vi "data collection.vi"(0 "Refnum in":T1, 1 "To Date":timestamp, 2 "Form Date":timestamp, 3 "Report filter":string, 5 "Shift":string, 7 "Select Line":string, 9 "Select Year":string, 11 "error in (no error)":errorcluster, 12 "columns":string[](array[string]), 13 "Select Month":string, 14 "table":string) -> (4 "Refnum out":T1, 6 "Table":string[][](array[string]), 8 "disabled index (col)":i32, 15 "error out":errorcluster)   [LabVIEW 2017]
uses:
  <vilib>/addons/database/Connection.llb/Conn ObjectReference.ctl
  <vilib>/addons/database/NI_Database_API.lvlib
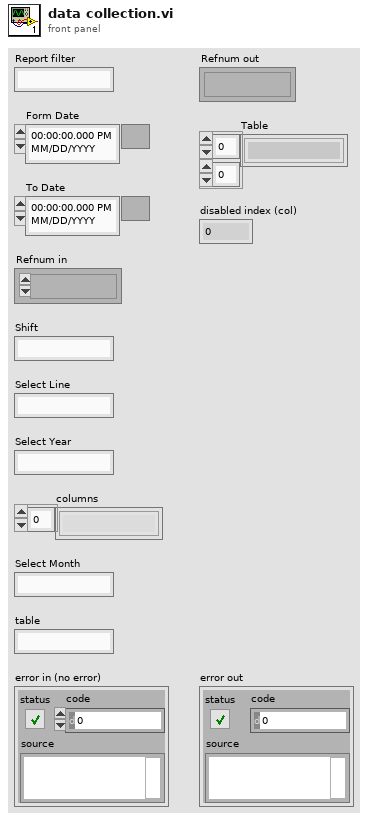
[diagram p1: front panel]
types:
  T1 = typedef "NI_Database_API.lvlib/Conn ObjectReference.ctl" = refnum<k1>
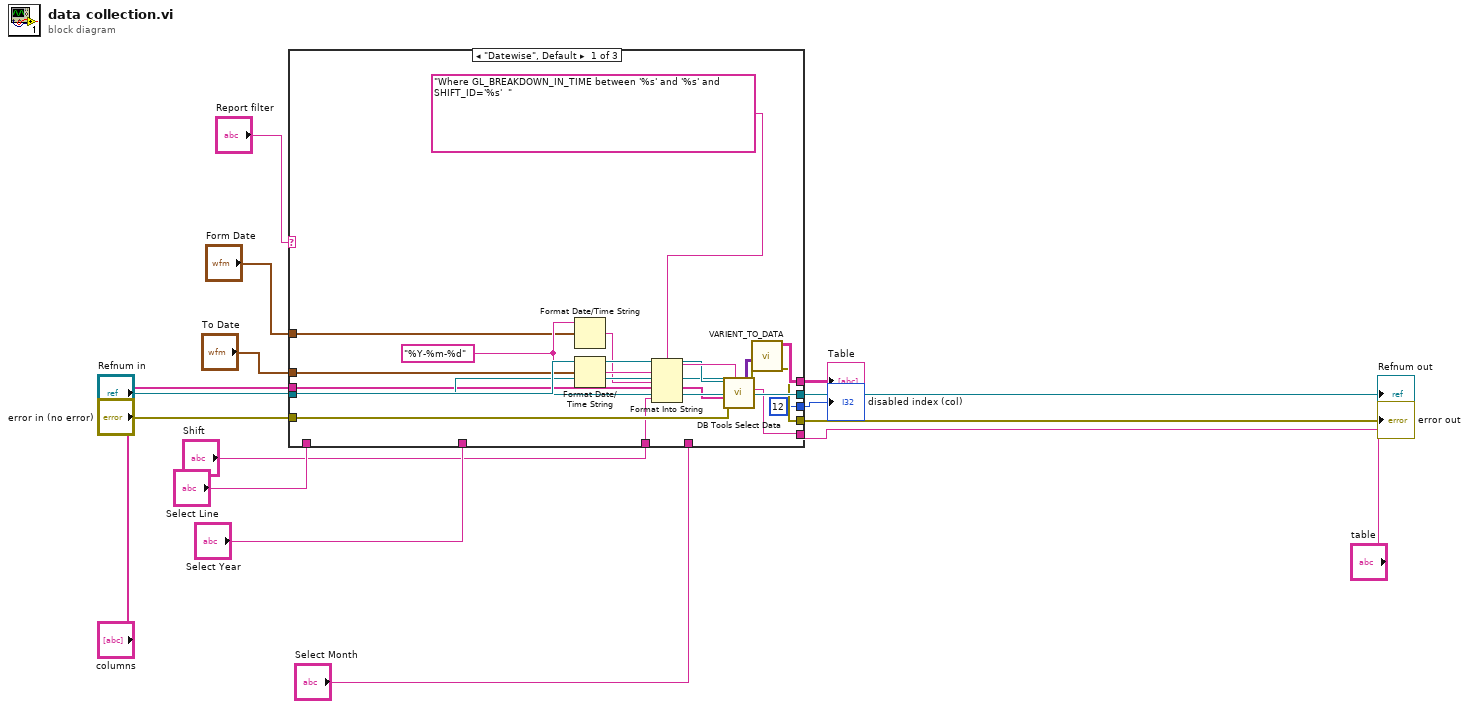
[diagram p0: block diagram]
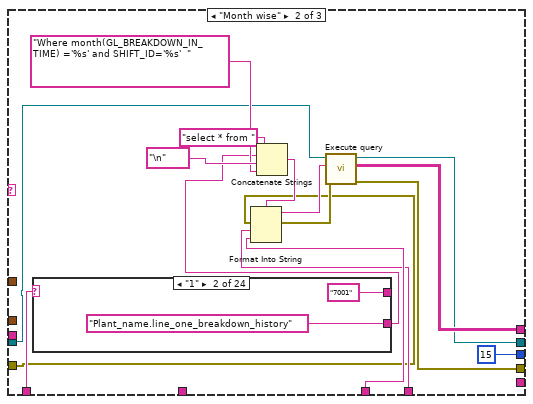
[diagram p2: hidden frame]
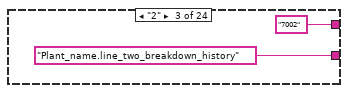
[diagram p4: hidden frame]
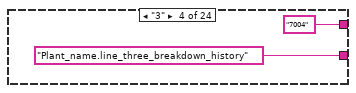
[diagram p5: hidden frame]
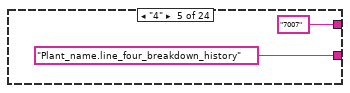
[diagram p6: hidden frame]
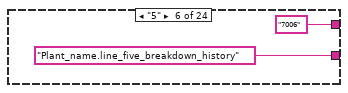
[diagram p7: hidden frame]
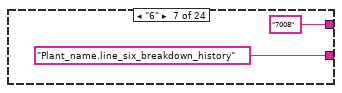
[diagram p8: hidden frame]
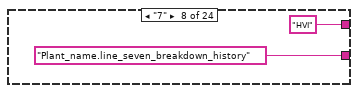
[diagram p9: hidden frame]
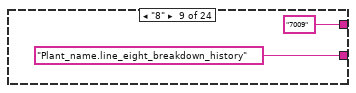
[diagram p10: hidden frame]
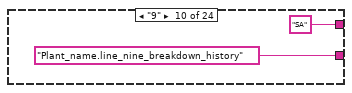
[diagram p11: hidden frame]
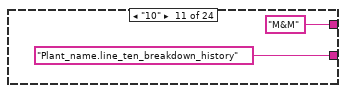
[diagram p12: hidden frame]
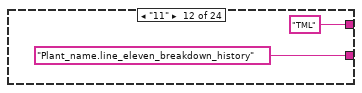
[diagram p13: hidden frame]
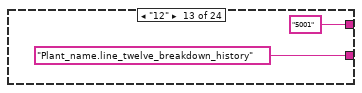
[diagram p14: hidden frame]
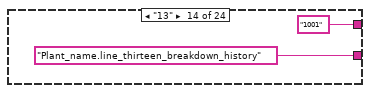
[diagram p15: hidden frame]
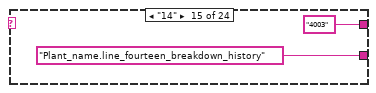
[diagram p16: hidden frame]
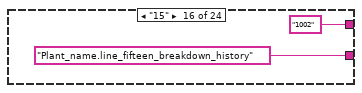
[diagram p17: hidden frame]
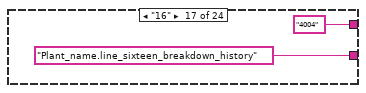
[diagram p18: hidden frame]
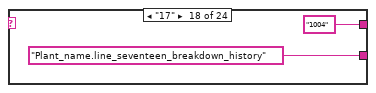
[diagram p19: hidden frame]
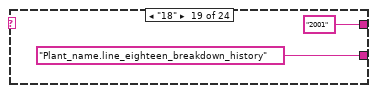
[diagram p20: hidden frame]
diagram:
  n1 = case shown="\"Datewise\", Default" "Report filter" {
    tunnel: [w31 w43 w106] -> w1
    tunnel: "Refnum in" -> [w30 w40 w103]
    tunnel: [w29 w42 w105] -> w3
    tunnel: "error in (no error)" -> [w28 w35 w99]
    tunnel: "table" -> [w27 _ _]
    tunnel: "columns" -> [w26 _ _]
    tunnel: [w24 w37 w101] -> w7
    tunnel: "Form Date" -> [w19 _ _]
    tunnel: "To Date" -> [w18 _ _]
    tunnel: "Shift" -> [w17 w39 w102]
    tunnel: "Select Line" -> [_ w45 w108]
    tunnel: "Select Month" -> [_ w38 _]
    tunnel: [12 ("disabled index (col)") 15 ("disabled index (col)") 15 ("disabled index (col)")] -> w14
    tunnel: "Select Year" -> [_ _ w96]
    frame "Datewise", Default {
      w23 = "%Y-%m-%d" ("time format string (%c)")
      n2 = Format Date/Time String(time format string (%c)=w23, seconds (now)=w19) -> (date/time string=w21:string)  [unwired: 1 in]
      n3 = Format Date/Time String(time format string (%c)=w23, seconds (now)=w18) -> (date/time string=w22:string)  [unwired: 1 in]
      n4 = Format Into String(format string="Where GL_BREAKDOWN_IN_TIME between '%s' and '%s' and SHIFT_ID='%s'  " ("condition"), w21, w22, w17) -> (resulting string=w33:string)  [unwired: 2 in, 1 out]
      n5 = call <vilib>:"DB Tools Select Data.vi"("condition"=w33, "error in (no error)"=w28, "columns"=w26, "table"=w27, "connection reference"=w30) -> ("error out"=w25:errorcluster, "data"=w32:variant[][], "connection reference out"=w29:T1)  [unwired: 1 in]
      n6 = call "VARIENT_TO_DATA.vi"("data"=w32, "error in (no error)"=w25) -> ("Table"=w31:string[][], "error out"=w24:errorcluster)  [unwired: 7 in]
    }
    frame "Month wise" {
      n7 = case shown="\"1\"" w45 {
        tunnel: [_ "7001" "7002" "7004" "7007" "7006" "7008" "HVI" "7009" "SA" "M&M" "TML" "5001" "1001" "4003" "1002" "4004" "1004" "2001" "3001" "2004" "3002" "3003" "4001"] -> _
        tunnel: [_ "Plant_name.line_one_breakdown_history" ("table") "Plant_name.line_two_breakdown_history" ("table") "Plant_name.line_three_breakdown_history" ("table") "Plant_name.line_four_breakdown_history" ("table") "Plant_name.line_five_breakdown_history" ("table") "Plant_name.line_six_breakdown_history" ("table") "Plant_name.line_seven_breakdown_history" ("table") "Plant_name.line_eight_breakdown_history" ("table") "Plant_name.line_nine_breakdown_history" ("table") "Plant_name.line_ten_breakdown_history" ("table") "Plant_name.line_eleven_breakdown_history" ("table") "Plant_name.line_twelve_breakdown_history" ("table") "Plant_name.line_thirteen_breakdown_history" ("table") "Plant_name.line_fourteen_breakdown_history" ("table") "Plant_name.line_fifteen_breakdown_history" ("table") "Plant_name.line_sixteen_breakdown_history" ("table") "Plant_name.line_seventeen_breakdown_history" ("table") "Plant_name.line_eighteen_breakdown_history" ("table") "Plant_name.line_nineteen_breakdown_history" ("table") "Plant_name.line_twenty_breakdown_history" ("table") "Plant_name.line_twenty_one_breakdown_history" ("table") "Plant_name.line_twenty_two_breakdown_history" ("table") "Plant_name.line_twenty_three_breakdown_history" ("table")] -> w44
        frame "0", Default {
        }
        frame "1" {
        }
        frame "2" {
        }
        frame "3" {
        }
        frame "4" {
        }
        frame "5" {
        }
        frame "6" {
        }
        frame "7" {
        }
        frame "8" {
        }
        frame "9" {
        }
        frame "10" {
        }
        frame "11" {
        }
        frame "12" {
        }
        frame "13" {
        }
        frame "14" {
        }
        frame "15" {
        }
        frame "16" {
        }
        frame "17" {
        }
        frame "18" {
        }
        frame "19" {
        }
        frame "20" {
        }
        frame "21" {
        }
        frame "22" {
        }
        frame "23" {
        }
      }
      n8 = Concatenate Strings("select * from " ("string"), w44, "\n" ("string"), "Where month(GL_BREAKDOWN_IN_TIME) ='%s' and SHIFT_ID='%s'  " ("condition")) -> (w46:string)
      n9 = Format Into String(format string=w46, error in=w35, w38, w39) -> (resulting string=w41:string, error out=w36:errorcluster)  [unwired: 1 in]
      n10 = call "Execute query.vi"("error in (no error)"=w36, "String"=w41, "connection reference"=w40) -> ("error out"=w37:errorcluster, "Table"=w43:string[][], "connection reference 2"=w42:T1)  [unwired: 5 in, 1 out]
    }
    frame "Year wise" {
      n11 = case shown="\"18\"" w108 {
        tunnel: [_ "7001" "7002" "7004" "7007" "7006" "7008" "HVI" "7009" "SA" "M&M" "TML" "5001" "1001" "4003" "1002" "4004" "1004" "2001" "3001" "2004" "3002" "3003" "4001"] -> _
        tunnel: [_ "Plant_name.line_one_breakdown_history" ("table") "Plant_name.line_two_breakdown_history" ("table") "Plant_name.line_three_breakdown_history" ("table") "Plant_name.line_four_breakdown_history" ("table") "Plant_name.line_five_breakdown_history" ("table") "Plant_name.line_six_breakdown_history" ("table") "Plant_name.line_seven_breakdown_history" ("table") "Plant_name.line_eight_breakdown_history" ("table") "Plant_name.line_nine_breakdown_history" ("table") "Plant_name.line_ten_breakdown_history" ("table") "Plant_name.line_eleven_breakdown_history" ("table") "Plant_name.line_twelve_breakdown_history" ("table") "Plant_name.line_thirteen_breakdown_history" ("table") "Plant_name.line_fourteen_breakdown_history" ("table") "Plant_name.line_fifteen_breakdown_history" ("table") "Plant_name.line_sixteen_breakdown_history" ("table") "Plant_name.line_seventeen_breakdown_history" ("table") "Plant_name.line_eighteen_breakdown_history" ("table") "Plant_name.line_nineteen_breakdown_history" ("table") "Plant_name.line_twenty_breakdown_history" ("table") "Plant_name.line_twenty_one_breakdown_history" ("table") "Plant_name.line_twenty_two_breakdown_history" ("table") "Plant_name.line_twenty_three_breakdown_history" ("table")] -> w107
        frame "0", Default {
        }
        frame "1" {
        }
        frame "2" {
        }
        frame "3" {
        }
        frame "4" {
        }
        frame "5" {
        }
        frame "6" {
        }
        frame "7" {
        }
        frame "8" {
        }
        frame "9" {
        }
        frame "10" {
        }
        frame "11" {
        }
        frame "12" {
        }
        frame "13" {
        }
        frame "14" {
        }
        frame "15" {
        }
        frame "16" {
        }
        frame "17" {
        }
        frame "18" {
        }
        frame "19" {
        }
        frame "20" {
        }
        frame "21" {
        }
        frame "22" {
        }
        frame "23" {
        }
      }
      n12 = Concatenate Strings("select * from " ("string"), w107, "\n" ("string"), "Where year(GL_BREAKDOWN_IN_TIME) ='%s' and SHIFT_ID='%s'  " ("condition")) -> (w109:string)
      n13 = Format Into String(format string=w109, error in=w99, w96, w102) -> (resulting string=w104:string, error out=w100:errorcluster)  [unwired: 1 in]
      n14 = call "Execute query.vi"("error in (no error)"=w100, "String"=w104, "connection reference"=w103) -> ("error out"=w101:errorcluster, "Table"=w106:string[][], "connection reference 2"=w105:T1)  [unwired: 5 in, 1 out]
    }
  }
  "disabled index (col)" <- w14
  "error out" <- w7
  "Refnum out" <- w3
  "Table" <- w1
